vi "Serialize - JSON.vi"(8 "error in":errorcluster, 11 "PPT Data in":refnum<class "PPT Data.lvclass">) -> (0 "error out":errorcluster, 2 "Serialized JSON":string, 3 "PPT Data out":refnum<class "PPT Data.lvclass">)   [LabVIEW 2014, in "PPT Library.lvlib" / "PPT Data.lvclass"]
uses:
  PPT Data.lvclass
  reusable/Data/Data.lvclass/Data.ctl
  PPT Data.lvclass/PPT Data.ctl
  reusable/Data/Read Data ID.vi
  Read P.vi
  Read T.vi
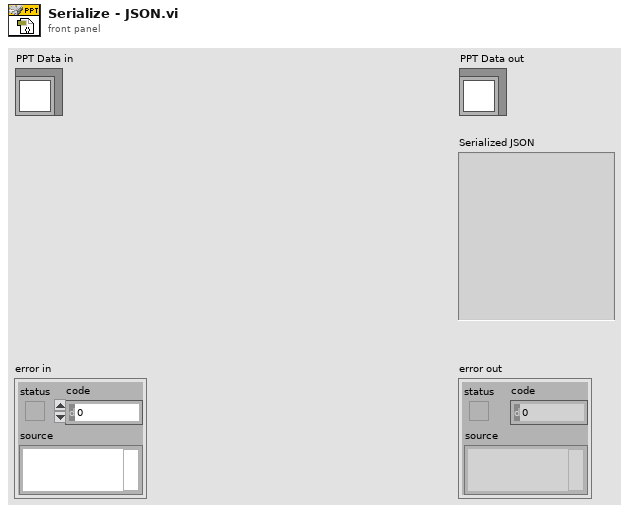
[diagram p1: front panel]
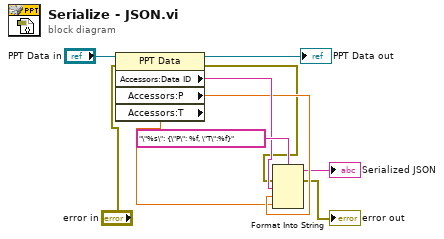
[diagram p0: block diagram]
diagram:
  n1 = property class="PPT Data"(reference="PPT Data in", error in="error in") -> (reference out=→"PPT Data out":refnum<class "PPT Data.lvclass">, error out=w2:errorcluster, "Accessors:Data ID"=w7:string, "Accessors:P"=w6:dbl, "Accessors:T"=w5:dbl)
  n2 = Format Into String(format string="\"%s\": {\"P\": %f, \"T\":%f}", error in=w2, w7, w6, w5) -> (resulting string=→"Serialized JSON":string, error out=→"error out":errorcluster)  [unwired: 1 in]
